vi "CheckCurrentLimits.vi"(11 "End Current":dbl) -> (3 "End Current":dbl)   [LabVIEW 2013]
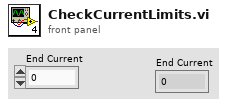
[diagram p1: front panel]
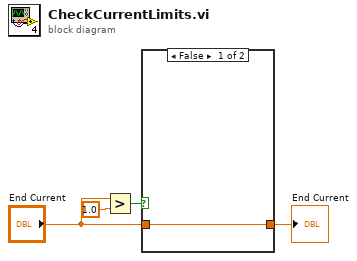
[diagram p0: block diagram]
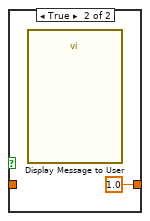
[diagram p2: hidden frame]
diagram:
  n1 = Greater?(x="End Current", y=1.0) -> (0:w3:bool)
  n2 = case shown="False" w3 {
    tunnel: [w5 1.0] -> w1
    tunnel: "End Current" -> [w5 _]
    frame False {
    }
    frame True {
      n3 = call "Display Message to User"() -> ()  [unwired: 10 in, 2 out]
    }
  }
  "End Current" <- w1
